vi "Initialize.vi"(7 "Serial Configuration":T1={"Baud Rate"=9600, "Parity"=0, "Data Bits"=8, "Stop Bits"=10, "Flow Control"=1} {"Flow Control" items=["None", "XON/XOFF", "RTS/CTS", "XON/XOFF & RTS/CTS", "DTR/DSR", "XON/XOFF & DTR/DSR"]; "Stop Bits" items=["1.0"=10, "1.5"=15, "2.0"=20]; "Data Bits" items=["7"=7, "8"=8]; "Parity" items=["None", "Odd", "Even", "Mark", "Space"]; "Baud Rate" items=["300"=300, "600"=600, "1200"=1200, "2400"=2400, "4800"=4800, "9600"=9600, "19200"=19200]}, 8 "error in (no error)":errorcluster, 9 "Reset (True)":bool=TRUE, 10 "ID Query (True)":bool=TRUE, 11 "VISA resource name":refnum<visa-resource-name>) -> (0 "error out":errorcluster, 3 "VISA resource name out":refnum<visa-resource-name>)   [LabVIEW 2015, in "Fluke 28x Series.lvlib"]
doc: "Establishes communication with the instrument and optionally performs an instrument identification query and/or an instrument reset. It also places the instrument in a default state needed for other instrument driver operations. Therefore, call this VI before calling other instrument driver VIs for this instrument. Generally, you need to call the Initialize VI only once at the beginning of an application.\n\n<b>Note</b>: VISA will return an error if the instrument is not explicitly set to communicate through GPIB. Use the Utility soft key and the Remote category to switch between serial and GPIB communication."
uses:
  <instrlib>/Fluke 28x Series/Fluke 28x Series.lvlib
panel:
  # "(c) 2009-2014 National Instruments.  ALL RIGHTS RESERVED."
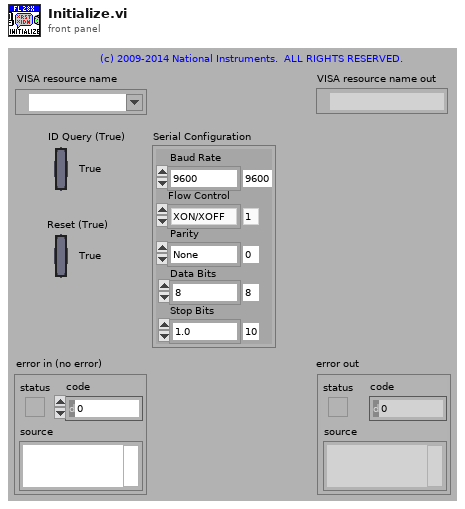
[diagram p1: front panel]
types:
  T1 = cluster{"Baud Rate":u32, "Parity":u16, "Data Bits":u16, "Stop Bits":u16, "Flow Control":u16}
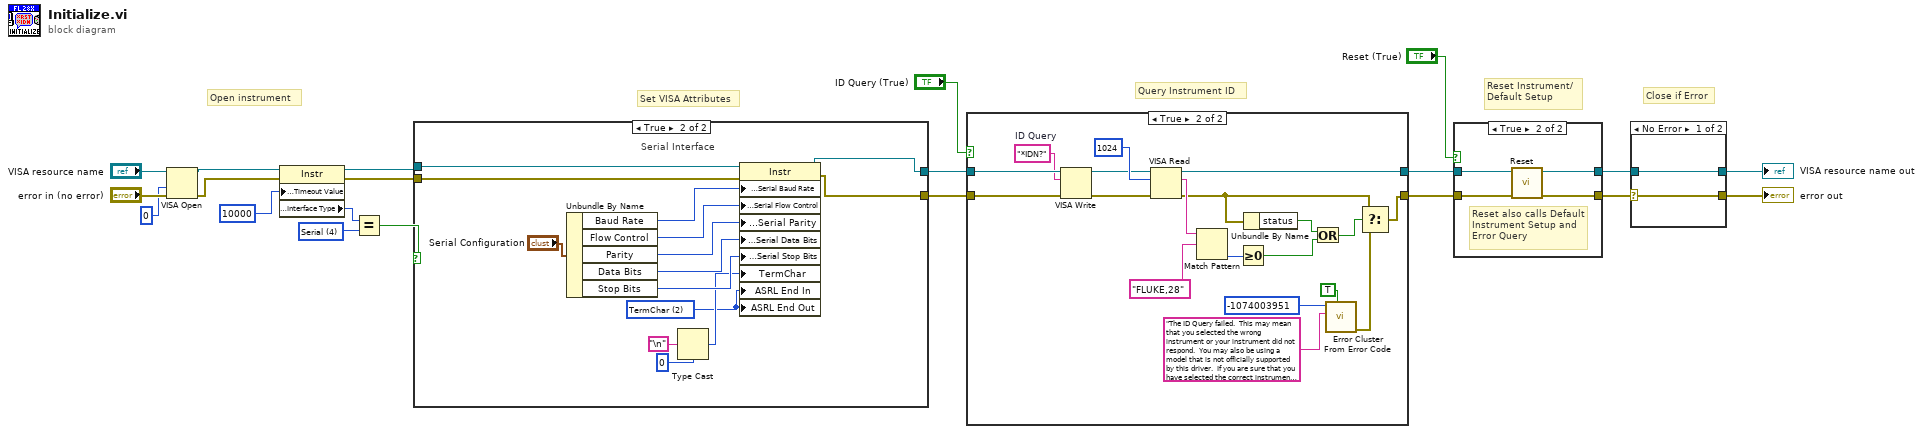
[diagram p0: block diagram]
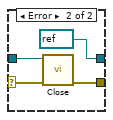
[diagram p3: hidden frame]
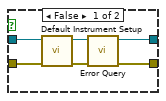
[diagram p4: hidden frame]
diagram:
  w6 = u16 4 items=["GPIB"=1, "VXI"=2, "GPIB-VXI"=3, "Serial"=4, "PXI"=5, "TCPIP"=6, "USB"=7] ("Interface Information:Interface Type")
  # "Set VISA Attributes"
  # "Close if Error"
  # "Query Instrument ID"
  # "Reset Instrument/\nDefault Setup"
  # "Open instrument"
  n1 = VISA Open(access mode=u32 0, error in (no error)="error in (no error)", VISA resource name="VISA resource name") -> (VISA resource name=w2:refnum<visa-resource-name>, error out=w1:errorcluster)  [unwired: 2 in]
  n2 = property class="Instr"(reference=w2, error in=w1, "General Settings:Timeout Value"=u32 10000) -> (reference out=w5:refnum<visa-resource-name>, error out=w4:errorcluster, "Interface Information:Interface Type"=w8:u16)
  n3 = Equal?(x=w8, y=w6) -> (x = y?=w3:bool)
  n4 = case shown="True" w3 {
    tunnel: [w23 w37] -> w15
    tunnel: [w22 w36] -> w14
    tunnel: w5 -> [w23 w25]
    tunnel: w4 -> [w22 w24]
    frame False {
      # "GPIB"
    }
    frame True {
      w26 = u16 2 items=["None", "LastBit", "TermChar"] ("Serial Settings:Serial End Mode for Reads")
      # "Serial Interface"
      n5 = Unbundle By Name("Serial Configuration") -> ("Baud Rate"=w35:u32, "Flow Control"=w32:u16, "Parity"=w33:u16, "Data Bits"=w34:u16, "Stop Bits"=w31:u16)
      n6 = Type Cast(type=u8 0, x="\n" ("Line Feed Constant")) -> (*(type *) &x=w27:u8)
      n7 = property class="Instr"(reference=w25, error in=w24, "Serial Settings:Serial Baud Rate"=w35, "Serial Settings:Serial Flow Control"=w32, "Serial Settings:Serial Parity"=w33, "Serial Settings:Serial Data Bits"=w34, "Serial Settings:Serial Stop Bits"=w31, "TermChar"=w27, "ASRL End In"=w26, "ASRL End Out"=w26) -> (reference out=w37:refnum<visa-resource-name>, error out=w36:errorcluster)
    }
  }
  n8 = case shown="True" "ID Query (True)" {
    tunnel: [w38 w58] -> w20
    tunnel: [w39 w55] -> w21
    tunnel: w15 -> [w39 w56]
    tunnel: w14 -> [w38 w57]
    frame False {
    }
    frame True {
      w42 = "*IDN?"  # ID Query
      n9 = VISA Write(VISA resource name=w56, write buffer=w42, error in (no error)=w57) -> (VISA resource name out=w41:refnum<visa-resource-name>, error out=w40:errorcluster)  [unwired: 1 out]
      n10 = VISA Read(VISA resource name=w41, byte count=u32 1024, error in (no error)=w40) -> (VISA resource name out=w55:refnum<visa-resource-name>, read buffer=w54:string, error out=w46:errorcluster)  [unwired: 1 out]
      n11 = Match Pattern(string=w54, regular expression="FLUKE,28") -> (offset past match=w47:i32)  [unwired: 1 in, 3 out]
      n12 = Greater Or Equal To 0?(x=w47) -> (x >= 0?=w44:bool)
      n13 = Unbundle By Name(w46) -> ("status"=w45:bool)
      n14 = Or(x=w45, y=w44) -> (x .or. y?=w43:bool)
      n15 = call <vilib>:"Error Cluster From Error Code.vi"("show call chain? (False)"=TRUE, "error message (\"\")"="The ID Query failed.  This may mean that you selected the wrong instrument or your instrument did not respond.  You may also be using a model that is not officially supported by this driver.  If you are sure that you have selected the correct instrument and it is responding, try disabling the ID Query." ("Source (VI Name)"), "error code (0)"=-1074003951 ("Code")) -> ("error out"=w51:errorcluster)  [unwired: 6 in]
      n16 = Select(t=w46, s=w43, f=w51) -> (s? t:f=w58:errorcluster)
    }
  }
  n17 = case shown="True" "Reset (True)" {
    tunnel: w20 -> [w63 w65]
    tunnel: [w60 w68] -> w9
    tunnel: w21 -> [w64 w66]
    tunnel: [w61 w67] -> w10
    frame False {
      n18 = call <instrlib>:"Default Instrument Setup.vi"("error in (no error)"=w63, "VISA resource name"=w64) -> ("error out"=w59:errorcluster, "VISA resource name out"=w62:refnum<visa-resource-name>)  [unwired: 8 in]
      n19 = call <instrlib>:"Error Query.vi"("error in (no error)"=w59, "VISA resource name"=w62) -> ("error out"=w60:errorcluster, "VISA resource name out"=w61:refnum<visa-resource-name>)  [unwired: 6 in, 2 out]
    }
    frame True {
      # "Reset also calls Default Instrument Setup and Error Query"
      n20 = call <instrlib>:"Reset.vi"("error in (no error)"=w65, "VISA resource name"=w66) -> ("error out"=w68:errorcluster, "VISA resource name out"=w67:refnum<visa-resource-name>)  [unwired: 8 in]
    }
  }
  n21 = case shown="No Error" w9 {
    selector: w9 -> [w69 w72]
    tunnel: w10 -> [w70 w73]
    tunnel: [w70 refnum<visa-resource-name> refnum ("VISA resource name out")] -> w12
    tunnel: [w69 w74] -> w11
    frame No Error {
    }
    frame Error {
      n22 = call <instrlib>:"Close.vi"("error in (no error)"=w72, "VISA resource name"=w73) -> ("error out"=w74:errorcluster)  [unwired: 9 in]
    }
  }
  "VISA resource name out" <- w12
  "error out" <- w11
